vi "Word_Insert_Table.vi"(0 "Document":refnum<k7>, 1 "Tables":refnum<k7>, 2 "font":T1 {"font size" format="%0.2f"; "strike through" items=["Unchanged", "Yes", "No"]; "underline" items=["Unchanged", "Yes", "No"]; "italic" items=["Unchanged", "Yes", "No"]; "bold" items=["Unchanged", "Yes", "No"]}, 3 "show grid lines":bool=TRUE, 5 "Table data":string[][](array[string]), 7 "Start":i32, 9 "End":i32, 11 "error in (no error)":errorcluster, 12 "Insertion point":u16(ring)=1 items=["begining of document", "end of document", "bookmark", "Custom"], 13 "Bookmark name":string, 14 "column width (1)":dbl format="%0.2f") -> (8 "Start out":i32, 10 "End out":i32, 15 "error out":errorcluster)   [LabVIEW 2017, in "NI_ReportGenerationToolkit.lvlib"]
uses:
  <vilib>/addons/_office/NI_ReportGenerationToolkit.lvlib
  <vilib>/addons/_office/_exclsub.llb/font.ctl
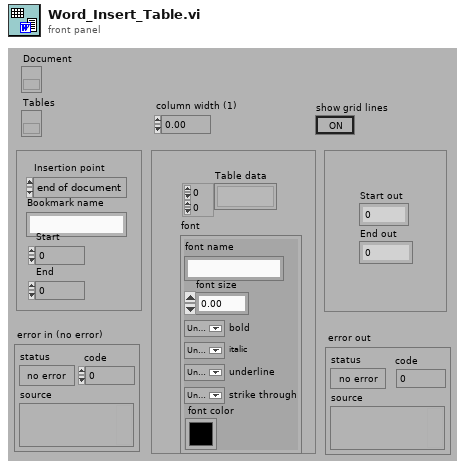
[diagram p1: front panel]
types:
  T1 = typedef "NI_ReportGenerationToolkit.lvlib/font.ctl" = cluster{"font name":string, "font size":dbl, "bold":u16, "italic":u16, "underline":u16, "strike through":u16, "font color":u32}
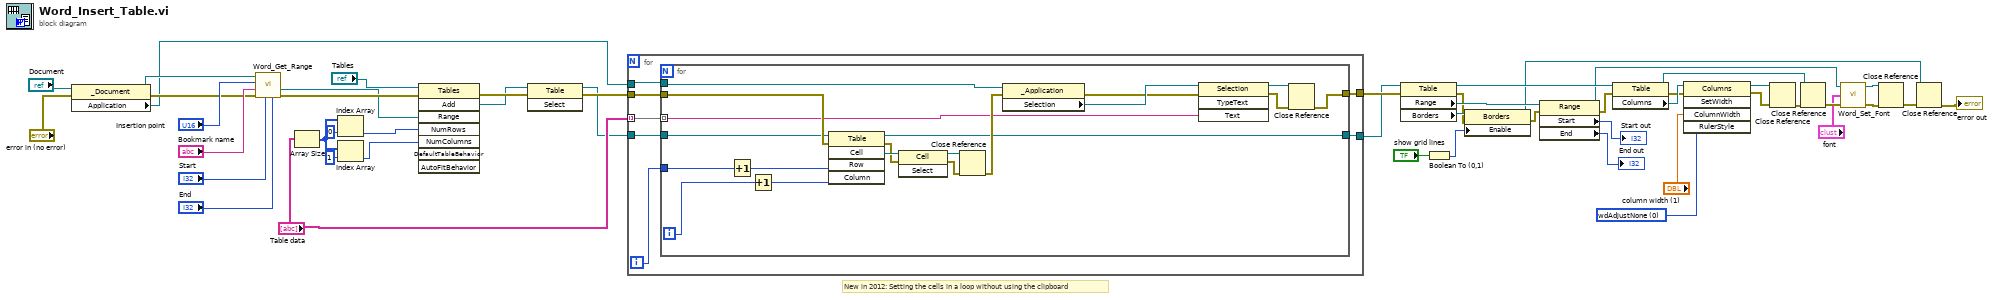
[diagram p0: block diagram]
diagram:
  w23 = 0 items=["wdAdjustNone", "wdAdjustProportional", "wdAdjustFirstColumn", "wdAdjustSameWidth"] ("RulerStyle")
  # "New in 2012: Setting the cells in a loop without using the clipboard"
  n1 = property class="_Document"(reference="Document", error in="error in (no error)") -> (reference out=w21:refnum<k7>, error out=w18:errorcluster, "Application"=w4:refnum<k7>)
  n2 = call <vilib>:"Word_Get_Range.vi"("end"="End", "start"="Start", "error in"=w18, "bookmark name"="Bookmark name", "insertion point"="Insertion point", "document in"=w21) -> ("error out (no error)"=w17:errorcluster, "range"=w16:refnum<k7>)  [unwired: 4 out]
  n3 = Array Size(array="Table data") -> (size(s)=w43:i32[])
  n4 = Index Array(array=w43, index=0 ("Indice")) -> (element=w40:i32)
  n5 = Index Array(array=w43, index=1 ("Indice")) -> (element=w39:i32)
  n6 = invoke class="Tables" method="Add"(reference="Tables", error in=w17, "Range"=w16, "NumRows"=w40, "NumColumns"=w39) -> (error out=w7:errorcluster, "Add"=w6:refnum<k7>)  [unwired: 3 in, 6 out]
  n7 = invoke class="Table" method="Select"(reference=w6, error in=w7) -> (reference out=w2:refnum<k7>, error out=w5:errorcluster)  [unwired: 1 in, 1 out]
  n8 = for {
    tunnel: "Table data" -> [w57] mode=indexing
    tunnel: [w56] -> w3
    tunnel: [w55] -> w8
    tunnel: w5 -> [w53]
    tunnel: w4 -> [w52]
    tunnel: w2 -> [w51]
    i -> [w54]
    n9 = for {
      tunnel: w57 -> [w67] mode=indexing
      tunnel: [w71] -> w56
      tunnel: [w64] -> w55
      tunnel: w54 -> [w63]
      tunnel: w53 -> [w70]
      tunnel: w52 -> [w69]
      tunnel: w51 -> [w68]
      i -> [w61]
      n10 = Increment(x=w63) -> (x+1=w62:i32)
      n11 = Increment(x=w61) -> (x+1=w60:i32)
      n12 = invoke class="Table" method="Cell"(reference=w68, error in=w70, "Row"=w62, "Column"=w60) -> (reference out=w71:refnum<k7>, error out=w75:errorcluster, "Cell"=w76:refnum<k7>)  [unwired: 1 in, 2 out]
      n13 = invoke class="Cell" method="Select"(reference=w76, error in=w75) -> (reference out=w72:refnum<k7>, error out=w74:errorcluster)  [unwired: 1 in, 1 out]
      n14 = Close Reference(reference=w72, error in (no error)=w74) -> (error out=w73:errorcluster)
      n15 = property class="_Application"(reference=w69, error in=w73) -> (error out=w58:errorcluster, "Selection"=w59:refnum<k7>)  [unwired: 1 out]
      n16 = invoke class="Selection" method="TypeText"(reference=w59, error in=w58, "Text"=w67) -> (reference out=w65:refnum<k7>, error out=w66:errorcluster)  [unwired: 1 in, 2 out]
      n17 = Close Reference(reference=w65, error in (no error)=w66) -> (error out=w64:errorcluster)
    }
  }
  n18 = property class="Table"(reference=w3, error in=w8) -> (reference out=w33:refnum<k7>, error out=w36:errorcluster, "Range"=w48:refnum<k7>, "Borders"=w37:refnum<k7>)
  n19 = Boolean To (0,1)(Boolean="show grid lines") -> (0, 1=w1:i16)
  n20 = property class="Borders"(reference=w37, error in=w36, "Enable"=w1) -> (reference out=w29:refnum<k7>, error out=w35:errorcluster)
  n21 = property class="Range"(reference=w48, error in=w35) -> (reference out=w12:refnum<k7>, error out=w32:errorcluster, "Start"=→"Start out":i32, "End"=→"End out":i32)
  n22 = property class="Table"(reference=w33, error in=w32) -> (reference out=w28:refnum<k7>, error out=w26:errorcluster, "Columns"=w27:refnum<k7>)
  n23 = invoke class="Columns" method="SetWidth"(reference=w27, error in=w26, "ColumnWidth"="column width (1)", "RulerStyle"=w23) -> (reference out=w30:refnum<k7>, error out=w25:errorcluster)  [unwired: 1 in, 3 out]
  n24 = Close Reference(reference=w30, error in (no error)=w25) -> (error out=w31:errorcluster)
  n25 = Close Reference(reference=w28, error in (no error)=w31) -> (error out=w15:errorcluster)
  n26 = call <vilib>:"Word_Set_Font.vi"("Range in"=w12, "font"="font", "Error in"=w15) -> ("Range out"=w11:refnum<k7>, "Error out"=w14:errorcluster)  [unwired: 5 out]
  n27 = Close Reference(reference=w11, error in (no error)=w14) -> (error out=w13:errorcluster)
  n28 = Close Reference(reference=w29, error in (no error)=w13) -> (error out=→"error out":errorcluster)
